vi "Romi-Drive-System-Act-OpenLoop.vi"(6 "Pass_Through_Time":dbl=-1.0 format="%33.4f", 8 "error in (no error)":errorcluster, 11 "RomiDriveDevRef":T1 {"GyroDevRef"."Sample Rate" min=0.25 max=100.0 step=0.25}) -> (0 "error out":errorcluster)   [LabVIEW 2019]
uses:
  Romi-Drive-System-Globals.vi
  <vilib>/Rock Robotics/WPI/ThirdParty/JAS_Junk/TrajLib/Trajectory_Library.lvlib
  <vilib>/Rock Robotics/SystemInterfaces/DIO/FPGA_DIOPWMChannel.ctl
  <vilib>/Rock Robotics/WPI/PWM/WPI_PWMDeadband.ctl
  <vilib>/Rock Robotics/WPI/MotorControl/WPI_MotorControlType.ctl
  <vilib>/Rock Robotics/SystemInterfaces/DIO/FPGA_DIOChannel.ctl
  <vilib>/Rock Robotics/WPI/MotorControl/WPI_MotorControlDeviceRef.ctl
  <vilib>/Rock Robotics/WPI/RobotDrive/WPI_RobotDriveDevRef.ctl
  <vilib>/Rock Robotics/SystemInterfaces/Encoder/FPGA_EncoderIdx.ctl
  <vilib>/Rock Robotics/WPI/Encoder/WPI_EncoderType.ctl
  <vilib>/Rock Robotics/SystemInterfaces/Counter/FPGA_CounterCtrSystemIndex.ctl
  <vilib>/Rock Robotics/WPI/Encoder/WPI_EncoderDevRef.ctl
  <vilib>/Rock Robotics/SystemInterfaces/spilib/spi_bus.ctl
  <vilib>/Rock Robotics/SystemInterfaces/AI/FPGA_AIChannel.ctl
  <vilib>/Rock Robotics/WPI/Gyro/WPI_GyroDevRef.ctl
  Romi-Drive-System-Device-Refs-TypeDef.ctl
panel:
  # "Analog"
  # "XRS"
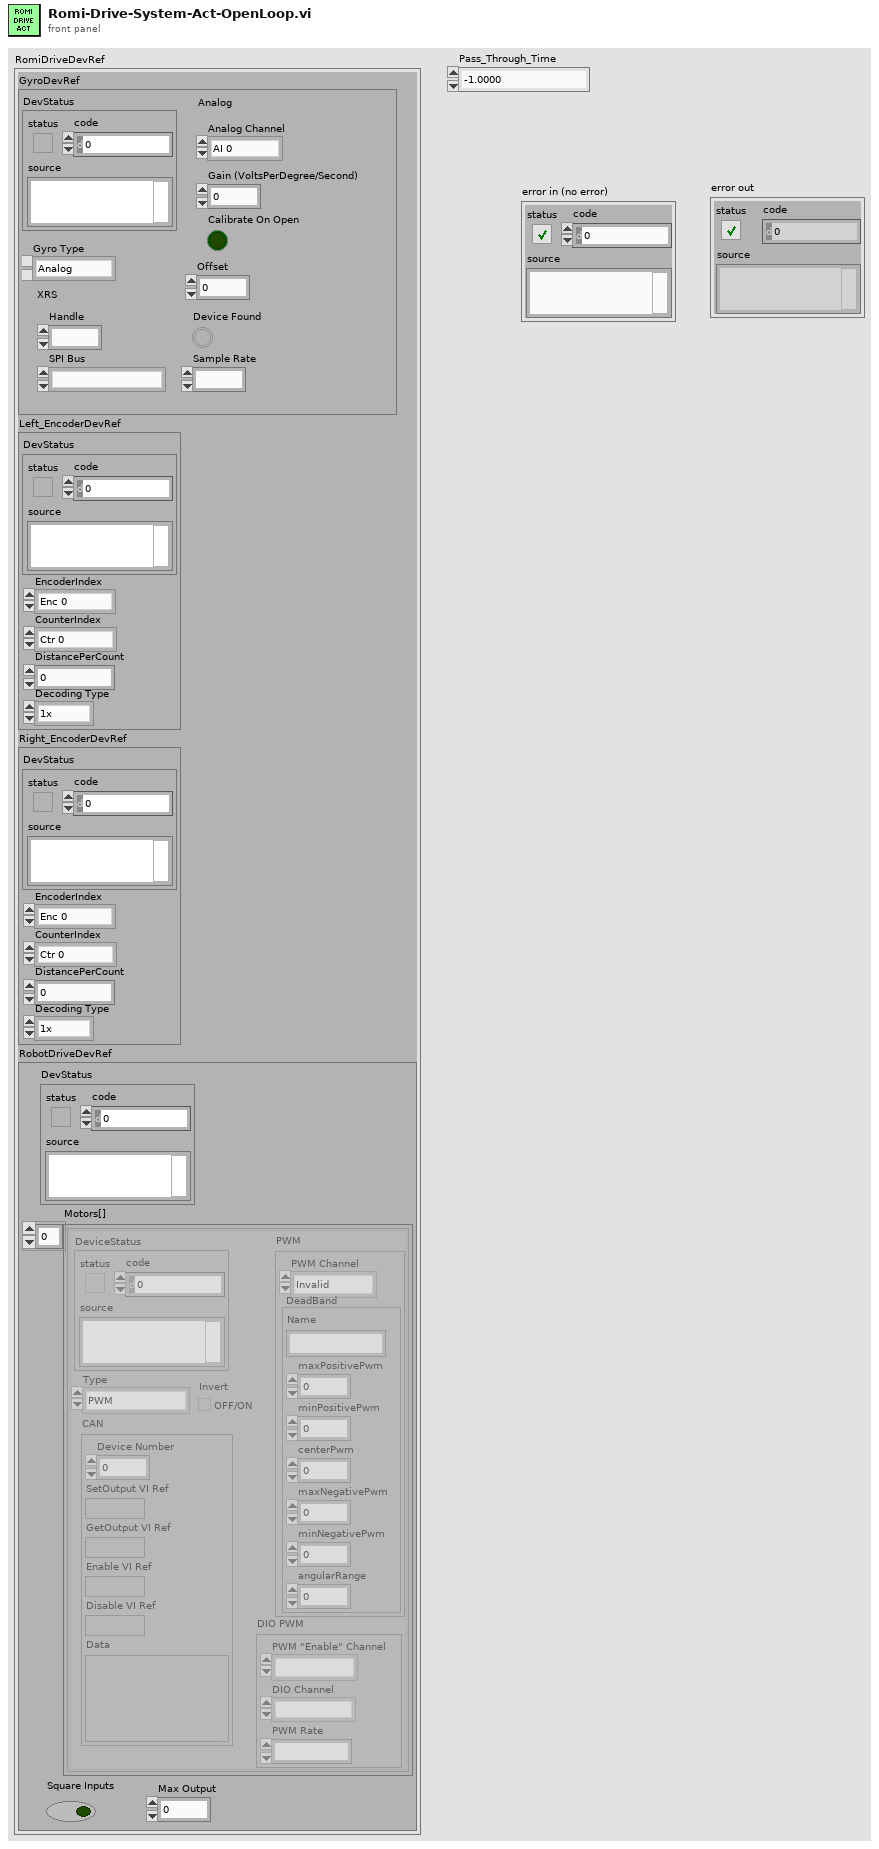
[diagram p1: front panel]
types:
  T1 = typedef "Romi-Drive-System-Device-Refs-TypeDef.ctl" = cluster{"GyroDevRef":T2, "Left_EncoderDevRef":T5, "Right_EncoderDevRef":T5, "RobotDriveDevRef":T9}
  T2 = typedef "WPI_GyroDevRef.ctl" = cluster{"DevStatus":errorcluster, "Analog Channel":T3, "Gain (VoltsPerDegree/Second)":dbl, "Gyro Type":enum16{"Analog", "XRS450"}, "Handle":i32, "SPI Bus":T4, "Device Found":bool, "Sample Rate":dbl, "Calibrate On Open":bool, "Offset":dbl}
  T3 = typedef "FPGA_AIChannel.ctl" = enum8{"AI 0", "AI 1", "AI 2", "AI 3", "AI MXP 0", "AI MXP 1", "AI MXP 2", "AI MXP 3", "Invalid"}
  T4 = typedef "spi_bus.ctl" = enum16{"SPI On-Board, CS0", "SPI On-Board, CS1", "SPI On-Board, CS2", "SPI On-Board, CS3", "SPI MXP", "Invalid"}
  T5 = typedef "WPI_EncoderDevRef.ctl" = cluster{"DevStatus":errorcluster, "EncoderIndex":T6, "CounterIndex":T7, "DistancePerCount":dbl, "Decoding Type":T8}
  T6 = typedef "FPGA_EncoderIdx.ctl" = enum8{"Enc 0", "Enc 1", "Enc 2", "Enc 3", "Enc 4", "Enc 5", "Enc 6", "Enc 7", "Invalid"}
  T7 = typedef "FPGA_CounterCtrSystemIndex.ctl" = enum8{"Ctr 0", "Ctr 1", "Ctr 2", "Ctr 3", "Ctr 4", "Ctr 5", "Ctr 6", "Ctr 7", "Invalid"}
  T8 = typedef "WPI_EncoderType.ctl" = enum16{"1x", "2x", "4x"}
  T9 = typedef "WPI_RobotDriveDevRef.ctl" = cluster{"DevStatus":errorcluster, "Motors[]":T10[], "Square Inputs":bool, "Max Output":dbl}
  T10 = typedef "WPI_MotorControlDeviceRef.ctl" = cluster{"DeviceStatus":errorcluster, "Type":T11, "PWM":cluster{"PWM Channel":T12, "DeadBand":T13}, "CAN":cluster{"Device Number":u8, "SetOutput VI Ref":variant, "GetOutput VI Ref":variant, "Enable VI Ref":variant, "Disable VI Ref":variant, "Data":variant}, "Invert":bool, "DIO PWM":cluster{"PWM \"Enable\" Channel":T12, "DIOChannel":T14, "PWM Rate":dbl}}
  T11 = typedef "WPI_MotorControlType.ctl" = enum16{"PWM", "CAN", "DIO PWM"}
  T12 = typedef "FPGA_DIOPWMChannel.ctl" = enum8{"PWM 0", "PWM 1", "PWM 2", "PWM 3", "PWM 4", "PWM 5", "PWM 6", "PWM 7", "PWM 8", "PWM 9", "PWM MXP 0", "PWM MXP 1", "PWM MXP 2", "PWM MXP 3", "PWM MXP 4", "PWM MXP 5", "PWM MXP 6", "PWM MXP 7", "PWM MXP 8", "PWM MXP 9", "Invalid"}
  T13 = typedef "WPI_PWMDeadband.ctl" = cluster{"Name":string, "maxPositivePwm":i32, "minPositivePwm":i32, "centerPwm":i32, "maxNegativePwm":i32, "minNegativePwm":i32, "angularRange":u16}
  T14 = typedef "FPGA_DIOChannel.ctl" = enum8{"DIO 0", "DIO 1", "DIO 2", "DIO 3", "DIO 4", "DIO 5", "DIO 6", "DIO 7", "DIO 8", "DIO 9", "DIO MXP 0", "DIO MXP 1", "DIO MXP 2", "DIO MXP 3", "DIO MXP 4", "DIO MXP 5", "DIO MXP 6", "DIO MXP 7", "DIO MXP 8", "DIO MXP 9", "DIO MXP 10", "DIO MXP 11", "DIO MXP 12", "DIO MXP 13", "DIO MXP 14", "DIO MXP 15", "SPI Port CS1", "SPI Port CS2", "SPI Port CS3", "SPI Port MISO", "SPI Port MOSI", "Invalid"}
  T15 = typedef "Trajectory_Library.lvlib/SIMPLE_MOTOR_FF.ctl" = cluster{"Ks":dbl, "Kv":dbl, "Ka":dbl, "KnInv":dbl}
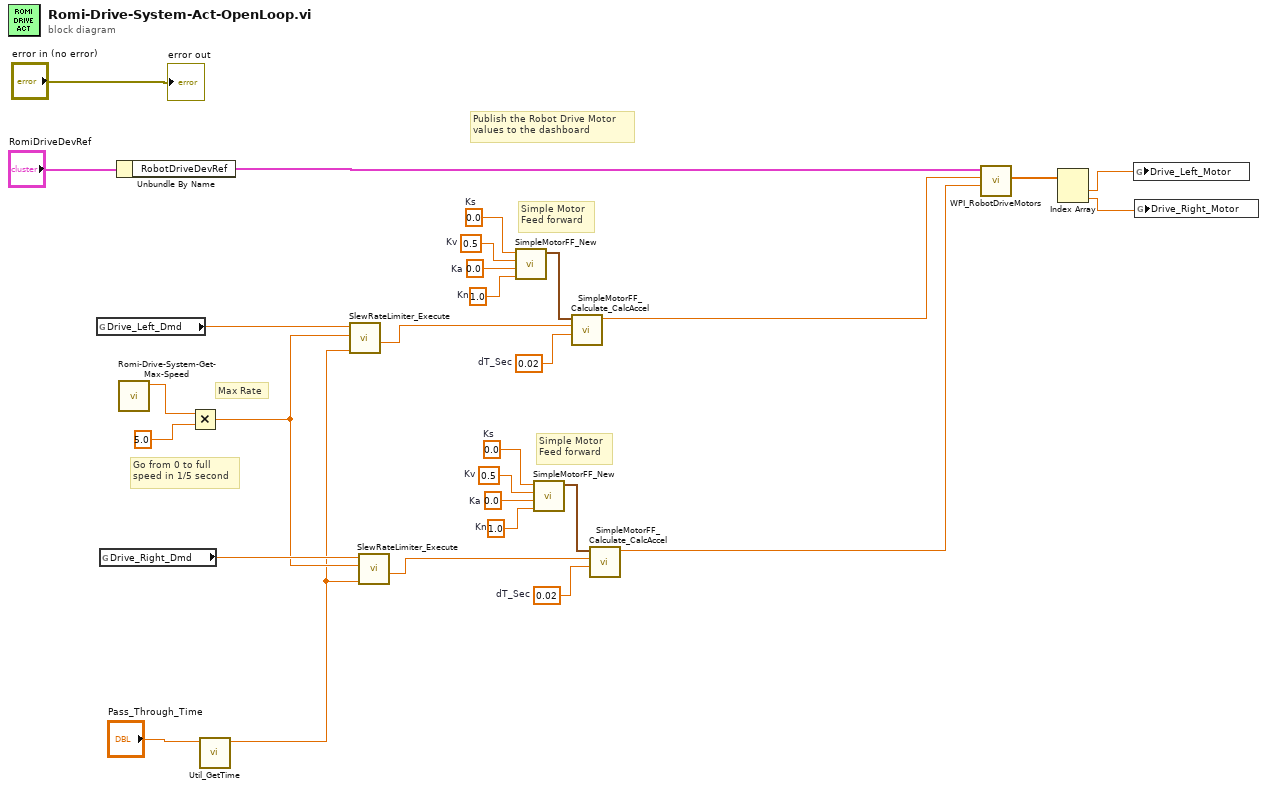
[diagram p0: block diagram]
diagram:
  w20 = 1.0  # Kn
  w19 = 0.02  # dT_Sec
  w17 = 0.0  # Ks
  w16 = 0.5  # Kv
  w15 = 0.0  # Ka
  w26 = 1.0  # Kn
  w25 = 0.02  # dT_Sec
  w23 = 0.0  # Ks
  w22 = 0.5  # Kv
  w21 = 0.0  # Ka
  # "Max Rate"
  # "Go from 0 to full \nspeed in 1/5 second"
  # "Simple Motor\nFeed forward"
  # "Simple Motor\nFeed forward"
  # "Publish the Robot Drive Motor\nvalues to the dashboard"
  n1 = global read "Romi-Drive-System-Globals.vi" "Drive_Left_Dmd"() -> (w7:dbl)
  n2 = global read "Romi-Drive-System-Globals.vi" "Drive_Right_Dmd"() -> (w4:dbl)
  n3 = Unbundle By Name("RomiDriveDevRef") -> ("RobotDriveDevRef"=w27:T9)
  n4 = call "Romi-Drive-System-Get-Max-Speed.vi"() -> ("MaxSpeed-Ft/Sec"=w9:dbl)  [unwired: 11 in]
  n5 = Multiply(x=w9, y=5.0) -> (x*y=w3:dbl)
  n6 = call <vilib>:"Util_GetTime.vi"("Pass_Through_Time"="Pass_Through_Time") -> ("FPGA_Time_Seconds"=w1:dbl)  [unwired: 9 in, 1 out]
  n7 = call <vilib>:"SlewRateLimiter_Execute.vi"("Time"=w1, "PositiveRate"=w3, "Input"=w7) -> ("Output"=w6:dbl)  [unwired: 7 in, 1 out]
  n8 = call <vilib>:"SlewRateLimiter_Execute.vi"("Time"=w1, "PositiveRate"=w3, "Input"=w4) -> ("Output"=w5:dbl)  [unwired: 7 in, 1 out]
  n9 = call <vilib>:"SimpleMotorFF_New.vi"("Kn"=w26, "Ka"=w21, "Kv"=w22, "Ks"=w23) -> ("SIMPLE_MOTOR_FF"=w24:T15)  [unwired: 7 in]
  n10 = call <vilib>:"SimpleMotorFF_New.vi"("Kn"=w20, "Ka"=w15, "Kv"=w16, "Ks"=w17) -> ("SIMPLE_MOTOR_FF"=w18:T15)  [unwired: 7 in]
  n11 = call <vilib>:"SimpleMotorFF_Calculate_CalcAccel.vi"("dT_Sec"=w25, "VelSp"=w6, "SIMPLE_MOTOR_FF"=w24) -> ("FeedForward"=w14:dbl)  [unwired: 8 in]
  n12 = call <vilib>:"SimpleMotorFF_Calculate_CalcAccel.vi"("dT_Sec"=w19, "VelSp"=w5, "SIMPLE_MOTOR_FF"=w18) -> ("FeedForward"=w13:dbl)  [unwired: 8 in]
  n13 = call <vilib>:"WPI_RobotDriveMotors.vi"("RightSpeed"=w13, "LeftSpeed"=w14, "RobotDriveDevRef"=w27) -> ("Motor Values"=w12:dbl[])  [unwired: 6 in, 2 out]
  n14 = Index Array(array=w12) -> (element #1=w11:dbl, element #2=w10:dbl)  [unwired: 2 in]
  n15 = global write "Romi-Drive-System-Globals.vi" "Drive_Left_Motor"(w11) -> ()
  n16 = global write "Romi-Drive-System-Globals.vi" "Drive_Right_Motor"(w10) -> ()
  "error out" <- "error in (no error)"
